vi "Parse Pinmap.vi"(8 "error in (no error)":errorcluster, 11 "Protocol Interface in":refnum<class "Protocol Interface.lvclass">) -> (0 "error out":errorcluster, 3 "Protocol Interface out":refnum<class "Protocol Interface.lvclass">)   [LabVIEW 2018]
uses:
  Protocol Interface.lvclass
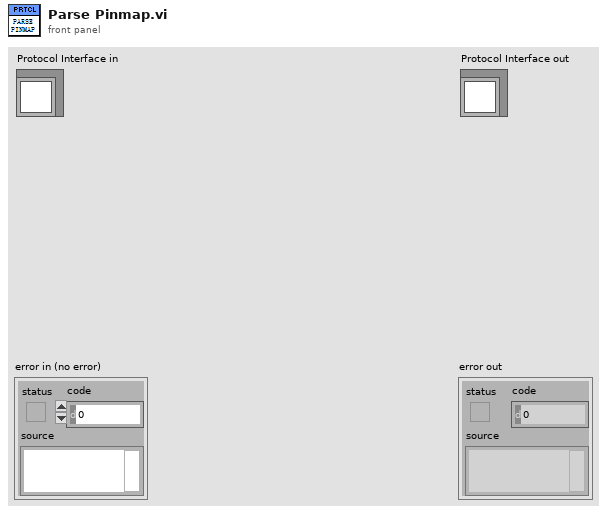
[diagram p1: front panel]
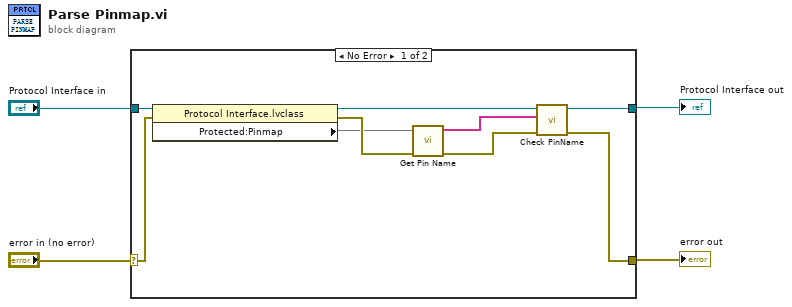
[diagram p0: block diagram]
diagram:
  n1 = case shown="No Error" "error in (no error)" {
    selector: "error in (no error)" -> [w12 w15]
    tunnel: [w9 w15] -> w3
    tunnel: [w10 w14] -> w1
    tunnel: "Protocol Interface in" -> [w13 w14]
    frame No Error {
      n2 = property class="Protocol Interface.lvclass"(reference=w13, error in=w12) -> (reference out=w11:refnum<class "Protocol Interface.lvclass">, error out=w6:errorcluster, "Protected:Pinmap"=w5)
      n3 = call "Get Pin Name.vi"("error in (no error)"=w6, "pin map"=w5) -> ("error out"=w7:errorcluster, "Pin Name"=w8:string[])  [unwired: 8 in]
      n4 = call-dynamic "Check PinName.vi"("error in (no error)"=w7, "Pin Array"=w8, "Protocol Interface in"=w11) -> ("error out"=w9:errorcluster, "Protocol Interface out"=w10:refnum<class "Protocol Interface.lvclass">)  [unwired: 7 in]
    }
    frame Error {
    }
  }
  "error out" <- w3
  "Protocol Interface out" <- w1
